vi "Read Color Area Size.vi"(8 "error in (no error)":errorcluster, 11 "ColorBox.lvclass in":refnum<class "ColorBox.lvclass">) -> (0 "error out":errorcluster, 2 "ColorAreaSize":T1, 3 "ColorBox.lvclass out":refnum<class "ColorBox.lvclass">)   [LabVIEW 2015, in "ColorBox.lvclass"]
uses:
  ColorBox.lvclass
  <vilib>/Utility/miscctls.llb/LVBoundsTypeDef.ctl
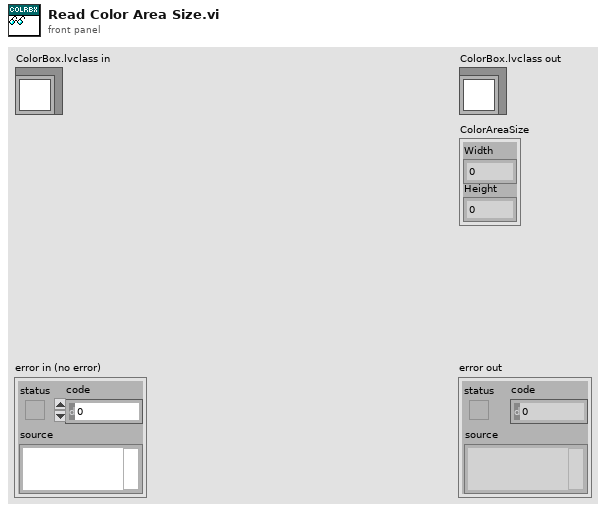
[diagram p1: front panel]
types:
  T1 = typedef "LVBoundsTypeDef.ctl" = cluster{"Width":u32, "Height":u32}
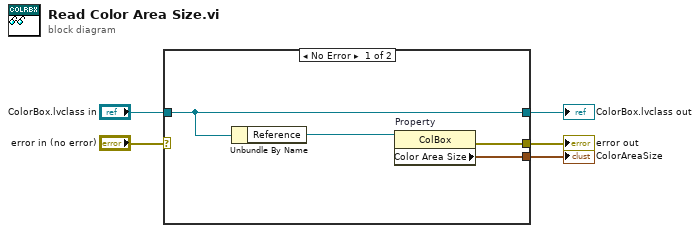
[diagram p0: block diagram]
diagram:
  n1 = case shown="No Error" "error in (no error)" {
    selector: "error in (no error)" -> [_ w11]
    tunnel: [w8 w11] -> w4
    tunnel: [w7 w10] -> w2
    tunnel: "ColorBox.lvclass in" -> [w7 w10]
    tunnel: [w9 _] -> w1
    frame No Error {
      n2 = Unbundle By Name(w7) -> ("Reference"=w6:refnum<vi>)
      n3 = property on="Property" class="ColBox"(reference=w6) -> (error out=w8:errorcluster, "Color Area Size"=w9:T1)  [unwired: 1 in, 1 out]
    }
    frame Error {
    }
  }
  "error out" <- w4
  "ColorBox.lvclass out" <- w2
  "ColorAreaSize" <- w1
